vi "Values on Tab Ctrl.vi"(6 "Max row":i32=15, 7 "Tab page Refnum":refnum<vi>, 8 "Error In":errorcluster, 9 "no. Rows":i32, 10 "Value":string[](array[string])) -> (0 "Error Out":errorcluster)   [LabVIEW 2014]
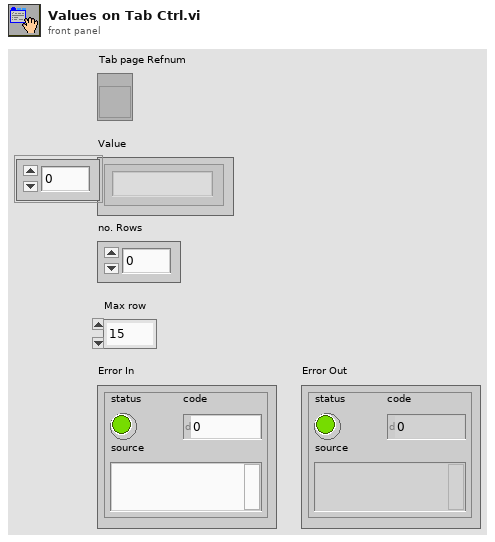
[diagram p1: front panel]
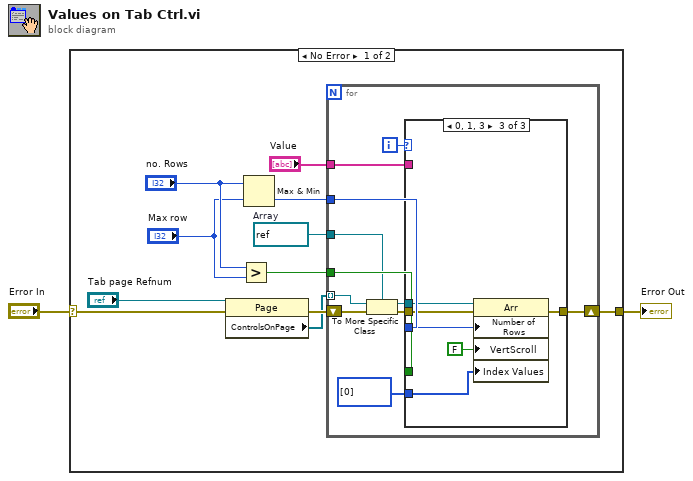
[diagram p0: block diagram]
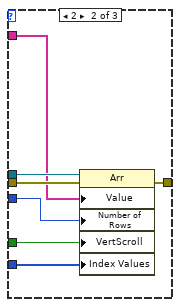
[diagram p3: hidden frame]
diagram:
  n1 = case shown="No Error" "Error In" {
    selector: "Error In" -> [w12 w39]
    tunnel: [w8 w39] -> w1
    frame No Error {
      w3 = refnum<vi> refnum  # Array
      n2 = property class="Page"(reference="Tab page Refnum", error in=w12) -> (error out=w10:errorcluster, "ControlsOnPage"=w4:refnum<vi>[])  [unwired: 1 out]
      n3 = Greater?(x="no. Rows", y="Max row") -> (0:w5:bool)
      n4 = Max & Min(x="no. Rows", y="Max row") -> (min(x,y)=w11:i32)  [unwired: 1 out]
      n5 = for {
        tunnel: w11 -> [w24]
        tunnel: "Value" -> [w20]
        tunnel: w5 -> [w18]
        shift-right: [w19] -> w8
        shift-left: w10 -> [w21]
        tunnel: w4 -> [w17] mode=indexing
        tunnel: w3 -> [w16]
        i -> [w15]
        n6 = To More Specific Class(target class=w16, reference=w17, error in=w21) -> (specific class reference=w22:refnum<vi>, error out=w23:errorcluster)
        n7 = case shown="0, 1, 3" w15 {
          tunnel: w24 -> [_ w32 w37]
          tunnel: w23 -> [w25 w31 w35]
          tunnel: w22 -> [_ w30 w36]
          tunnel: w20 -> [_ w29 _]
          tunnel: [w25 w28 w34] -> w19
          tunnel: w18 -> [_ w27 _]
          tunnel: u32[] [0] ("Index Values") -> [_ w26 w33]
          frame -1, Default {
          }
          frame 2 {
            n8 = property class="Arr"(reference=w30, error in=w31, "Value"=w29, "Number of Rows"=w32, "VertScroll"=w27, "Index Values"=w26) -> (error out=w28:errorcluster)  [unwired: 1 out]
          }
          frame 0, 1, 3 {
            n9 = property class="Arr"(reference=w36, error in=w35, "Number of Rows"=w37, "VertScroll"=FALSE ("Vertical Scrollbar Visible"), "Index Values"=w33) -> (error out=w34:errorcluster)  [unwired: 1 out]
          }
        }
      }
    }
    frame Error {
    }
  }
  "Error Out" <- w1
